vi "niFpgaIPINodeSimWrapper.vi"   [LabVIEW 2017]
uses:
  <vilib>/rvi/IPIntegrationNode/IPINode_Typedef/niFpgaIPINodeSupportedFamilies.ctl
types:
  T1 = typedef "niFpgaIPINodeSupportedFamilies.ctl" = cluster{"unlimited?":bool, "supported targets":string[]}
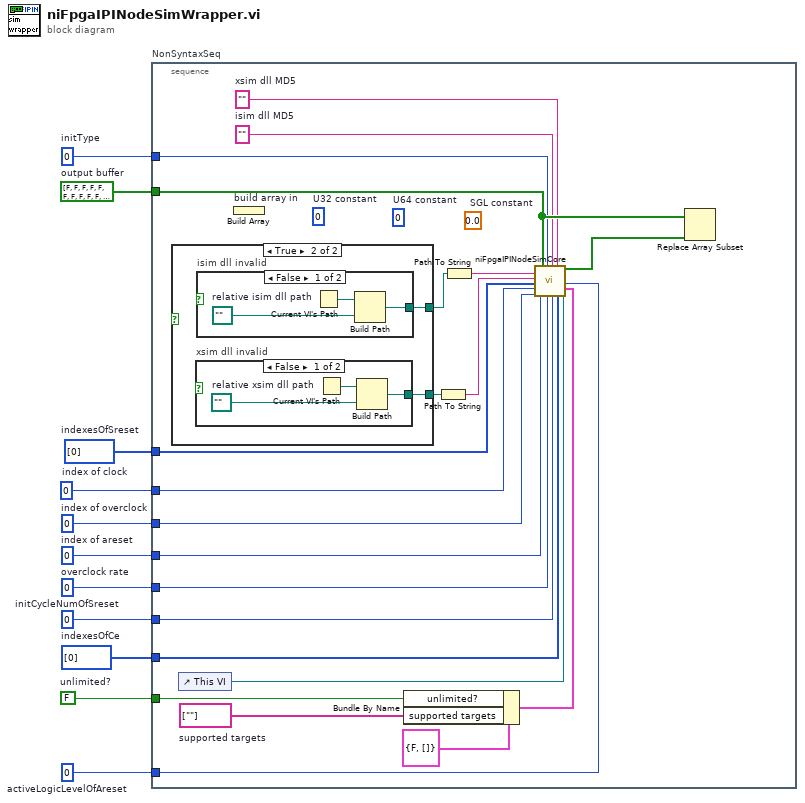
[diagram p0: block diagram]
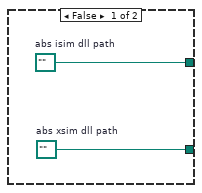
[diagram p2: hidden frame]
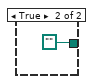
[diagram p3: hidden frame]
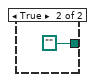
[diagram p4: hidden frame]
diagram:
  w1 = u8 0  # activeLogicLevelOfAreset
  w2 = FALSE  # unlimited?
  w3 = i32[] [0]  # indexesOfCe
  w4 = i32[] [0]  # indexesOfSreset
  w5 = u16 0  # initType
  w6 = 0  # initCycleNumOfSreset
  w7 = 0  # index of overclock
  w8 = 0  # overclock rate
  w9 = bool[] [FALSE, FALSE, FALSE, FALSE, FALSE, FALSE, FALSE, FALSE, FALSE, FALSE, FALSE, FALSE, FALSE, FALSE, FALSE, FALSE, FALSE, FALSE, FALSE]  # output buffer
  w10 = 0  # index of areset
  w11 = 0  # index of clock
  n1 = stacked-sequence "NonSyntaxSeq" {
    tunnel: w11 -> [w26]
    tunnel: w10 -> [w24]
    tunnel: w9 -> [w33]
    tunnel: w8 -> [w23]
    tunnel: w7 -> [w25]
    tunnel: w6 -> [w22]
    tunnel: w5 -> [w29]
    tunnel: w4 -> [w27]
    tunnel: w3 -> [w21]
    tunnel: w2 -> [w15]
    tunnel: w1 -> [w12]
    frame #0 {
      w14 = string[] [""]  # supported targets
      w19 = ""  # xsim dll MD5
      w28 = ""  # isim dll MD5
      (unwired) sgl 0.0  # SGL constant
      (unwired) u64 0  # U64 constant
      (unwired) u32 0  # U32 constant
      n2 = case shown="True" {
        selector: _ -> [_ _]
        tunnel: [w35 w37] -> w31
        tunnel: [w34 w36] -> w18
        frame False {
          w34 = path ""  # abs xsim dll path
          w35 = path ""  # abs isim dll path
        }
        frame True {
          n3 = case "xsim dll invalid" shown="False" {
            selector: _ -> [_ _]
            tunnel: [w38 path ""] -> w36
            frame False {
              w39 = path ""  # relative xsim dll path
              n4 = Current VI's Path() -> (path=w40:path)
              n5 = Build Path(base path=w40, name or relative path=w39) -> (appended path=w38:path)
            }
            frame True {
            }
          }
          n6 = case "isim dll invalid" shown="False" {
            selector: _ -> [_ _]
            tunnel: [w42 path ""] -> w37
            frame False {
              w43 = path ""  # relative isim dll path
              n7 = Current VI's Path() -> (path=w44:path)
              n8 = Build Path(base path=w44, name or relative path=w43) -> (appended path=w42:path)
            }
            frame True {
            }
          }
        }
      }
      n9 = control-ref of="This VI"() -> (w17:refnum<vi>)
      n10 = Build Array "build array in"() -> ()  [unwired: 1 in, 1 out]
      n11 = Bundle By Name(cluster=T1 {"unlimited?"=FALSE, "supported targets"=[]} ("targets"), "unlimited?"=w15, "supported targets"=w14) -> (w13:T1)
      n12 = Path To String(path=w18) -> (string=w20:string)
      n13 = Path To String(path=w31) -> (string=w30:string)
      n14 = call <vilib>:"niFpgaIPINodeSimCore.vi"("isim dll path"=w30, "xsim dll path"=w20, "indexesOfSreset"=w27, "index of clock"=w26, "indexOfOverclock"=w25, "outputs in"=w33, "index of areset"=w24, "initType"=w29, "overclockRate"=w23, "isim dll MD5"=w28, "initCycleNumOfSreset"=w22, "xsim dll MD5"=w19, "indexesOfCe"=w21, "activeLogicLevelOfAreset"=w12, "targets"=w13, "owning VI Ref"=w17) -> ("outputs"=w32:bool[])  [unwired: 3 in]
      n15 = Replace Array Subset "replace array subset"(array=w33, new element=w32) -> ()  [unwired: 1 in, 1 out]
    }
  }
